vi "pixel to stage coordinates.vi"(8 "Slide (mm)":T1={"top"=-12.263, "right"=-22.214, "width"=60.0, "height"=25.4}, 9 "Y in (px)":i32, 10 "X in (px)":i32) -> (1 "Y out (mm)":dbl, 2 "X out (mm)":dbl)   [LabVIEW 2023]
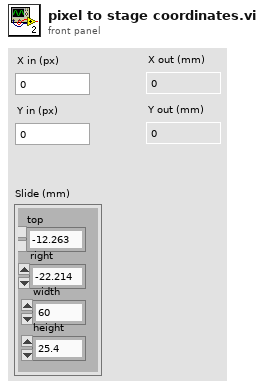
[diagram p1: front panel]
types:
  T1 = cluster{"top":dbl, "right":dbl, "width":dbl, "height":dbl}
  T2 = typedef "imagedata.ctl" = cluster{"image type":i32, "image depth":i32, "image":u8[], "mask":u8[], "colors":u32[], "Rectangle":cluster{"left":i16, "top":i16, "right":i16, "bottom":i16}}
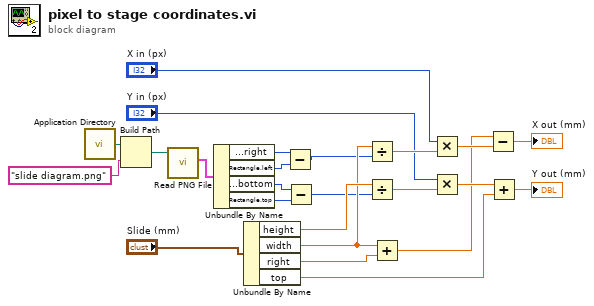
[diagram p0: block diagram]
diagram:
  n1 = call <vilib>:"Application Directory.vi"() -> ("Application Directory"=w10:path)
  n2 = Build Path(base path=w10, name or relative path="slide diagram.png") -> (appended path=w9:path)
  n3 = call <vilib>:"Read PNG File.vi"("path to PNG file"=w9) -> ("image data"=w8:T2)  [unwired: 8 in, 2 out]
  n4 = Unbundle By Name(w8) -> ("Rectangle.right"=w7:i16, "Rectangle.left"=w6:i16, "Rectangle.bottom"=w5:i16, "Rectangle.top"=w4:i16)
  n5 = Unbundle By Name("Slide (mm)") -> ("height"=w24:dbl, "width"=w12:dbl, "right"=w13:dbl, "top"=w18:dbl)
  n6 = Subtract(x=w7, y=w6) -> (x-y=w3:i16)
  n7 = Subtract(x=w5, y=w4) -> (x-y=w2:i16)
  n8 = Divide(x=w12, y=w3) -> (x/y=w22:dbl)
  n9 = Divide(x=w24, y=w2) -> (x/y=w21:dbl)
  n10 = Add(x=w12, y=w13) -> (x+y=w14:dbl)
  n11 = Multiply(x="X in (px)", y=w22) -> (x*y=w16:dbl)
  n12 = Multiply(x="Y in (px)", y=w21) -> (x*y=w19:dbl)
  n13 = Subtract(x=w14, y=w16) -> (x-y=→"X out (mm)":dbl)
  n14 = Add(x=w19, y=w18) -> (x+y=→"Y out (mm)":dbl)
